vi "Update Alias Endpoint.vi"(6 "Previous Alias":string, 8 "error in (no error)":errorcluster, 9 "Endpoint":string, 10 "Alias":string, 11 "Aliases Ref in":T1 format="%.0x") -> (0 "error out":errorcluster, 3 "Aliases Ref out":T1 format="%.0x")   [LabVIEW 2020, in "Routing and Faulting System Explorer.lvlib"]
uses:
  Routing and Faulting System Explorer.lvlib
  <vilib>/NI VeriStand/Custom Device API/Custom Device Item Ref.ctl
  Parse Endpoint.vi
  Scripting/Routing and Faulting Scripting.lvlib
  <vilib>/NI VeriStand/Custom Device API/Custom Device API.lvlib
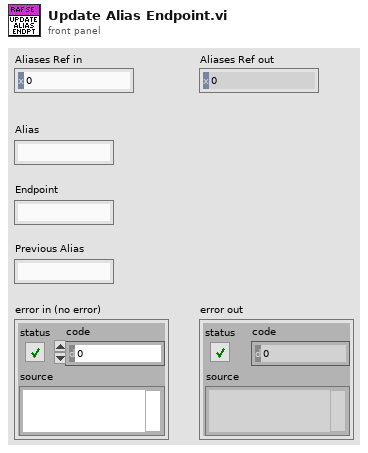
[diagram p1: front panel]
types:
  T1 = typedef "Custom Device API.lvlib/Custom Device Item Ref.ctl" = u64
  T2 = typedef "Routing and Faulting Shared.lvlib/Alias Endpoint.ctl" = cluster{"Module Path":string, "Endpoint":string}
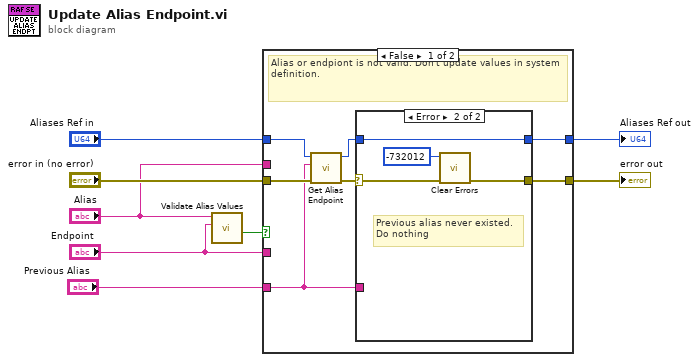
[diagram p0: block diagram]
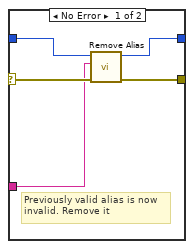
[diagram p2: hidden frame]
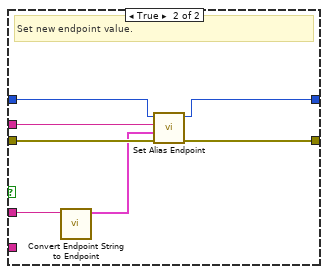
[diagram p3: hidden frame]
diagram:
  n1 = call "Validate Alias Values.vi"("Endpoint"="Endpoint", "Alias"="Alias") -> ("Valid"=w2:bool)  [unwired: 8 in, 1 out]
  n2 = case shown="False" w2 {
    tunnel: "Alias" -> [_ w31]
    tunnel: "Endpoint" -> [_ w26]
    tunnel: "Aliases Ref in" -> [w14 w27]
    tunnel: "error in (no error)" -> [w15 w30]
    tunnel: [w11 w29] -> w6
    tunnel: [w10 w28] -> w5
    tunnel: "Previous Alias" -> [w9 _]
    frame False {
      # "Alias or endpiont is not valid. Don't update values in system definition."
      n3 = call "Get Alias Endpoint.vi"("error in"=w15, "alias"=w9, "endpoint aliases in"=w14) -> ("error out"=w13:errorcluster, "endpoint aliases out"=w12:T1)  [unwired: 6 in, 1 out]
      n4 = case shown="Error" w13 {
        selector: w13 -> [w20 w23]
        tunnel: w12 -> [w19 w21]
        tunnel: [w18 w22] -> w11
        tunnel: [w17 w21] -> w10
        tunnel: w9 -> [w16 _]
        frame No Error {
          # "Previously valid alias is now\ninvalid. Remove it"
          n5 = call "Remove Alias.vi"("error in"=w20, "alias"=w16, "endpoint aliases in"=w19) -> ("error out"=w18:errorcluster, "endpoint aliases out"=w17:T1)  [unwired: 7 in]
        }
        frame Error {
          # "Previous alias never existed.\nDo nothing"
          n6 = call <vilib>:"Clear Errors.vi"("error in (no error)"=w23, "specific error code to clear (0: all)"=-732012) -> ("error out"=w22:errorcluster)  [unwired: 4 in, 1 out]
        }
      }
    }
    frame True {
      # "Set new endpoint value."
      n7 = call "Convert Endpoint String to Endpoint.vi"("Endpoint String"=w26) -> ("Endpoint"=w25:T2)  [unwired: 10 in]
      n8 = call "Set Alias Endpoint.vi"("error in"=w30, "new endpoint"=w25, "alias"=w31, "endpoint aliases in"=w27) -> ("error out"=w29:errorcluster, "endpoint aliases out"=w28:T1)  [unwired: 6 in]
    }
  }
  "Aliases Ref out" <- w5
  "error out" <- w6
